vi "Write Topic Lookup Table.vi"(8 "error in (no error)":errorcluster, 10 "TopicLookupTable":refnum<data-value>, 11 "MediatorBusMonitor in":refnum<class "MediatorBusMonitor.lvclass">) -> (0 "error out":errorcluster, 3 "MediatorBusMonitor out":refnum<class "MediatorBusMonitor.lvclass">)   [LabVIEW 2015, in "Mediator.lvlib" / "MediatorBusMonitor.lvclass"]
uses:
  MediatorBusMonitor.lvclass
  TopicLookupTable/TopicLookupTable.lvclass
  MediatorBusMonitor.lvclass/MediatorBusMonitor.ctl
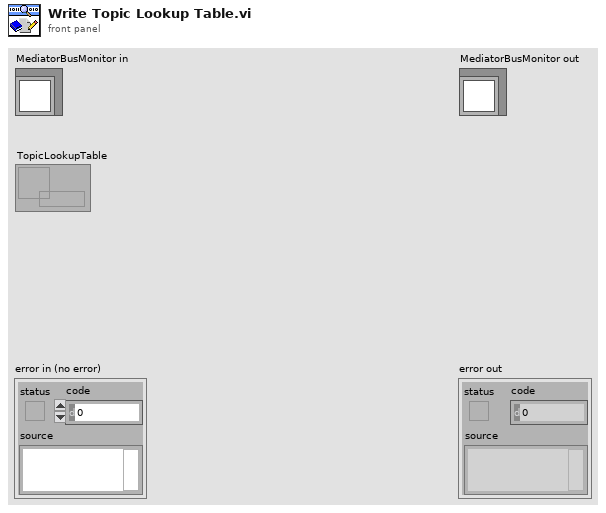
[diagram p1: front panel]
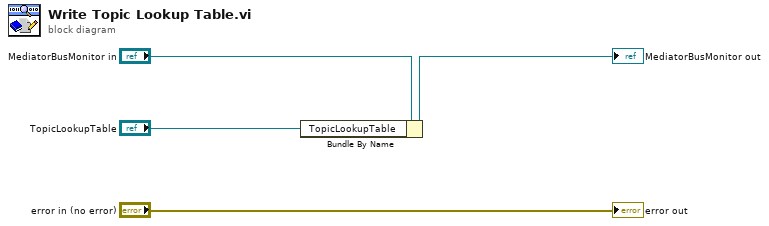
[diagram p0: block diagram]
diagram:
  n1 = Bundle By Name(cluster="MediatorBusMonitor in", "TopicLookupTable"="TopicLookupTable") -> (→"MediatorBusMonitor out":refnum<class "MediatorBusMonitor.lvclass">)
  "error out" <- "error in (no error)"
